vi "FXP Filtered-X LMS.vi"(7 "reset":bool, 9 "step size":fxp<+/-,16,-2> caption="mu", 10 "e(n)":fxp<+/-,24,4>, 11 "x(n)":fxp<+/-,24,4>) -> (3 "y(n)":fxp<+/-,24,4>)   [LabVIEW 2023]
uses:
  <vilib>/Utility/error.llb/Clear Errors.vi
  <vilib>/rvi/Emulation/niFpgaSctlEmulationGetInTimedLoop.vi
  <vilib>/rvi/Memory/Memory_Emulation/nirvimemoryEmulation.vi
  <vilib>/rvi/Memory/Memory_Emulation/nirvimemoryFastEmulation.vi
  <vilib>/rvi/DataTransferAndStorage/Container/Common/niFpgaContainerGetUniqueNameForEmu.vi
  <vilib>/rvi/Memory/Memory_Emulation/niFpgaMemoryEmulationCacheClearOnFirstRun.vi
  <vilib>/rvi/Memory/Memory_Emulation/nirvimemoryEmulationManagerCache_MakeExclusive.vi
  <vilib>/rvi/Memory/Memory_Emulation/niFpgaMemoryEmulationValidateCache.vi
  <vilib>/rvi/Memory/Memory_Emulation/nirvimemoryEmulationManagerCache_InsertValue.vi
  <vilib>/rvi/Memory/Memory_Emulation/nirvimemoryEmulationManagerCache_ReleaseExclusive.vi
  <vilib>/rvi/Memory/Memory_Emulation/nirvimemoryEmulationManagerCache_GetValue.vi
  <vilib>/rvi/Emulation/niFpgaEmulationIsFPGAContextNoSignature.vi
  <vilib>/rvi/Memory/Memory_Emulation/nirvimemoryEmulationManagerCache_SetValue.vi
  <vilib>/rvi/Emulation/niFpgaSctlEmulationResourceMgr.vi
  <vilib>/rvi/DataTransferAndStorage/Container/Common/niFpgaContainerSetEmuInfo.vi
  <vilib>/rvi/eio/common/nirviEmuReportErrorAndStop.vi
  <vilib>/rvi/DataTransferAndStorage/Container/XNode/niFpgaContainer.xnode
  <vilib>/rvi/FXPMathLib/FxpMul/XNode/nifxpmath_Multiplier.xnode
  <vilib>/rvi/FXPMathLib/FxpAdd/XNode/nifxpmath_Add.xnode
  <vilib>/rvi/FXPMathLib/FxpSub/XNode/nifxpmath_Sub.xnode
  <vilib>/rvi/LocalResourceManager/LocalResourceManager.xnode
  <vilib>/rvi/FXPMathLib/sim/FxpSim.dll
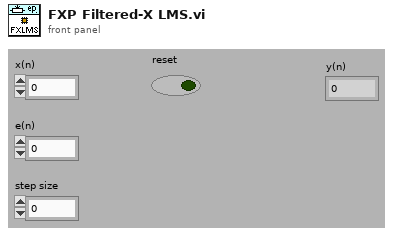
[diagram p1: front panel]
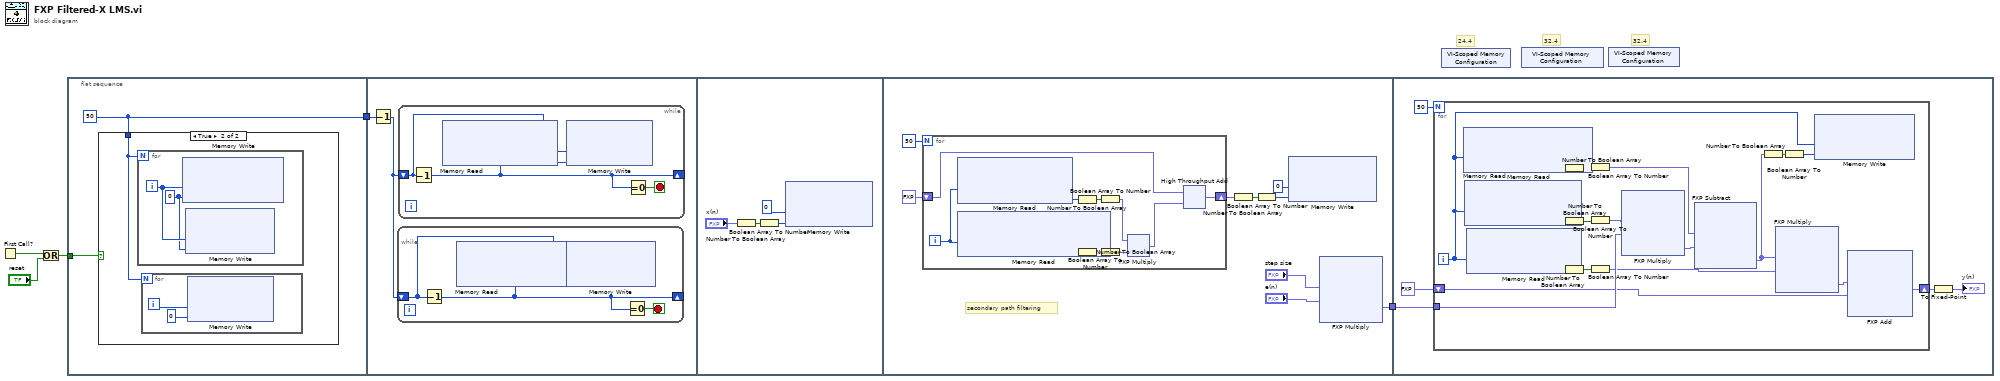
[diagram p0: block diagram]
diagram:
  # "32.4"
  # "32.4"
  # "24.4"
  n1 = First Call?() -> (First Call?: T/F=w3:bool)
  n2 = Or(x=w3, y="reset") -> (x .or. y?=w2:bool)
  n3 = flat-sequence {
    tunnel: [w6] -> w5
    tunnel: w2 -> [w7]
    tunnel: w5 -> [w14]
    tunnel: [w29] -> w1
    tunnel: w1 -> [w49]
    frame #0 {
      w6 = 50
      n4 = case shown="True" w7 {
        tunnel: w6 -> [_ w8]
        frame False {
        }
        frame True {
          n5 = for {
            N: w8 -> [_]
            i -> [w12]
            w11 = 0
            n6 = xnode ("Memory Write")("Address"=w12, "Data"=w11) -> ()  [unwired: 1 in, 1 out]
            n7 = xnode ("Memory Write")("Address"=w12, "Data"=w11) -> ()  [unwired: 1 in, 1 out]
          }
          n8 = for {
            N: w8 -> [_]
            i -> [w10]
            n9 = xnode ("Memory Write")("Address"=w10, "Data"=i16 0) -> ()  [unwired: 1 in, 1 out]
          }
        }
      }
    }
    frame #1 {
      n10 = Decrement(x=w14) -> (x-1=w13:i32)
      n11 = while {
        shift-right: [w17] -> _
        shift-left: w13 -> [w16]
        stop <- w18 stop-if-true
        n12 = Decrement(x=w16) -> (x-1=w17:i32)
        n13 = xnode ("Memory Read")("Address"=w17) -> ("Data"=w15:i32)  [unwired: 1 in, 1 out]
        n14 = xnode ("Memory Write")("Address"=w16, "Data"=w15) -> ()  [unwired: 1 in, 1 out]
        n15 = Equal To 0?(x=w17) -> (x = 0?=w18:bool)
      }
      n16 = while {
        shift-right: [w21] -> _
        shift-left: w13 -> [w20]
        stop <- w22 stop-if-true
        n17 = Decrement(x=w20) -> (x-1=w21:i32)
        n18 = xnode ("Memory Read")("Address"=w21) -> ("Data"=w19:i32)  [unwired: 1 in, 1 out]
        n19 = xnode ("Memory Write")("Address"=w20, "Data"=w19) -> ()  [unwired: 1 in, 1 out]
        n20 = Equal To 0?(x=w21) -> (x = 0?=w22:bool)
      }
    }
    frame #2 {
      n21 = Number To Boolean Array(number="x(n)") -> (Boolean array=w24:bool[])
      n22 = Boolean Array To Number(Boolean array=w24) -> (number=w23:i32)
      n23 = xnode ("Memory Write")("Address"=u32 0, "Data"=w23) -> ()  [unwired: 1 in, 1 out]
    }
    frame #3 {
      # "secondary path filtering"
      n24 = for {
        N: 50 -> [_]
        shift-right: [w37] -> w27
        shift-left: fxp<+/-,32,4> 0.0 ("x+y") -> [w38]
        i -> [w45]
        n25 = xnode ("Memory Read")("Address"=w45) -> ("Data"=w41:i32)  [unwired: 1 in, 1 out]
        n26 = xnode ("Memory Read")("Address"=w45) -> ("Data"=w43:fxp<+/-,24,4>)  [unwired: 1 in, 1 out]
        n27 = Number To Boolean Array(number=w41) -> (Boolean array=w42:bool[])
        n28 = Number To Boolean Array(number=w43) -> (Boolean array=w44:bool[])
        n29 = Boolean Array To Number(Boolean array=w42) -> (number=w39:fxp<+/-,24,4>)
        n30 = Boolean Array To Number(Boolean array=w44) -> (number=w40:fxp<+/-,24,4>)
        n31 = xnode "FXP Multiply"("x"=w39, "y"=w40) -> ("x*y"=w36:fxp<+/-,32,4>)
        n32 = xnode "High Throughput Add"("x"=w38, "y"=w36) -> ("x+y"=w37:fxp<+/-,32,4>)
      }
      n33 = Number To Boolean Array(number=w27) -> (Boolean array=w33:bool[])
      n34 = Boolean Array To Number(Boolean array=w33) -> (number=w32:i32)
      n35 = xnode ("Memory Write")("Address"=u32 0, "Data"=w32) -> ()  [unwired: 1 in, 1 out]
      n36 = xnode "FXP Multiply"("x"="step size", "y"="e(n)") -> ("x*y"=w29:fxp<+/-,32,2>)
    }
    frame #4 {
      n37 = for {
        N: 50 -> [_]
        shift-right: [w56] -> w48
        shift-left: fxp<+/-,32,4> 0.0 ("n") -> [w55]
        tunnel: w49 -> [w63]
        i -> [w68]
        n38 = xnode ("Memory Read")("Address"=w68) -> ("Data"=w66:i32)  [unwired: 1 in, 1 out]
        n39 = xnode ("Memory Read")("Address"=w68) -> ("Data"=w64:i32)  [unwired: 1 in, 1 out]
        n40 = xnode ("Memory Read")("Address"=w68) -> ("Data"=w58:i32)  [unwired: 1 in, 1 out]
        n41 = Number To Boolean Array(number=w66) -> (Boolean array=w67:bool[])
        n42 = Number To Boolean Array(number=w64) -> (Boolean array=w65:bool[])
        n43 = Number To Boolean Array(number=w58) -> (Boolean array=w59:bool[])
        n44 = Boolean Array To Number(Boolean array=w67) -> (number=w53:fxp<+/-,32,4>)
        n45 = Boolean Array To Number(Boolean array=w65) -> (number=w62:fxp<+/-,32,4>)
        n46 = Boolean Array To Number(Boolean array=w59) -> (number=w57:fxp<+/-,24,4>)
        n47 = xnode "FXP Multiply"("x"=w62, "y"=w63) -> ("x*y"=w52:fxp<+/-,32,4>)
        n48 = xnode "FXP Subtract"("x"=w53, "y"=w52) -> ("x-y"=w51:fxp<+/-,32,4>)
        n49 = Number To Boolean Array(number=w51) -> (Boolean array=w61:bool[])
        n50 = xnode "FXP Multiply"("x"=w51, "y"=w57) -> ("x*y"=w54:fxp<+/-,32,4>)
        n51 = Boolean Array To Number(Boolean array=w61) -> (number=w60:i32)
        n52 = xnode ("Memory Write")("Address"=w68, "Data"=w60) -> ()  [unwired: 1 in, 1 out]
        n53 = xnode "FXP Add"("x"=w54, "y"=w55) -> ("x+y"=w56:fxp<+/-,32,4>)
      }
      n54 = To Fixed-Point(number=w48) -> (fixed-point=→"y(n)":fxp<+/-,24,4>)  [unwired: 1 out]
    }
  }
  n55 = xnode "VI-Scoped Memory Configuration"() -> ()  [unwired: 1 out]
  n56 = xnode "VI-Scoped Memory Configuration"() -> ()  [unwired: 1 out]
  n57 = xnode "VI-Scoped Memory Configuration"() -> ()  [unwired: 1 out]
